vi "Sym Encoder 16 2.vi"   [LabVIEW 2013]
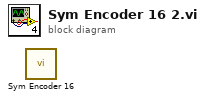
[diagram p0: block diagram]
diagram:
  n1 = call "Sym Encoder 16.vi"() -> ()  [unwired: 11 in, 1 out]
